vi "Set Dual Exposure Times.vi"(8 "error in (no error)":errorcluster, 10 "expTime2":sgl, 11 "expTime1":sgl) -> (0 "error out":errorcluster, 3 "function return":u32)   [LabVIEW 2014, in "atmcd32d.lvlib"]
doc: "unsigned int WINAPI SetDualExposureTimes(float expTime1, float expTime2);"
uses:
  atmcd32d.lvlib
  atmcd32d.dll
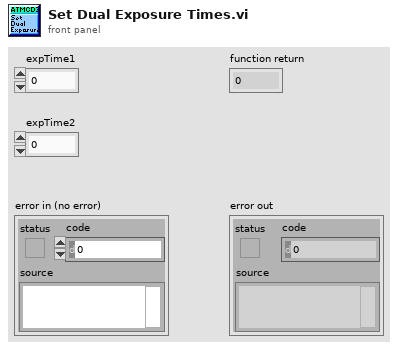
[diagram p1: front panel]
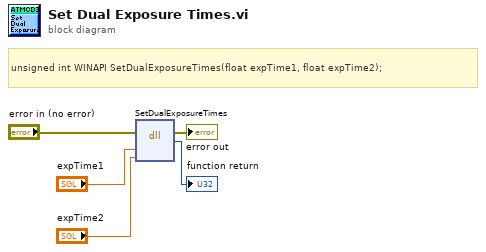
[diagram p0: block diagram]
diagram:
  # "unsigned int WINAPI SetDualExposureTimes(float expTime1, float expTime2);"
  n1 = dll-call lib="C:/Users/Bakir/Documents/Lambda2-Testing/lib/Andorlib/atmcd32d.*" fn="SetDualExposureTimes"(error in="error in (no error)", "expTime1"="expTime1", "expTime2"="expTime2") -> (error out=→"error out":errorcluster, →"function return":u32)  [unwired: 4 in, 1 out]
